vi "Initialize Queue.vi"(8 "error in":errorcluster) -> (0 "error out":errorcluster, 3 "Queue out":refnum<queue>)   [LabVIEW 2020, in "MHL.lvlib"]
doc: "Initialize Enqueue and Dequeue FGV and send message with the initializer state for the state machine.\n\n--------------------\nJuan Navarro\nLab It Studio"
uses:
  MHL.lvlib
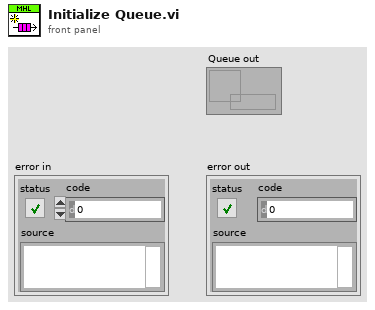
[diagram p1: front panel]
types:
  T1 = enum16{"Obtain", "Enqueue", "Get Queue", "Flush", "Release"}
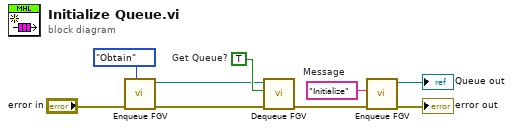
[diagram p0: block diagram]
diagram:
  w9 = TRUE  # Get Queue?
  w4 = "Initialize"  # Message
  n1 = call "Enqueue FGV.vi"("Actions"=T1."Obtain", "error in"="error in") -> ("error out"=w7:errorcluster, "queue out"=w6:refnum<queue>)  [unwired: 8 in]
  n2 = call "Dequeue FGV.vi"("error in"=w7, "Get Queue?"=w9, "queue in"=w6) -> ("error out"=w8:errorcluster)  [unwired: 5 in, 3 out]
  n3 = call "Enqueue FGV.vi"("error in"=w8, "Message"=w4) -> ("error out"=→"error out":errorcluster, "queue out"=→"Queue out":refnum<queue>)  [unwired: 8 in]
